vi "ma_Process RMS for 1 Block.vi"(6 "reset":bool, 7 "window for RMS":T2(ring)=enum."Hanning", 8 "time signal data (samples)":dbl[](array[numeric]) format="%0.2p", 10 "averaging type":enum16{"Linear", "Exponential"}(ring), 11 "state info":T1 {"buffer" format="%0.2f"; "timestamp" format="%<%.4X>T"; "dt history" format="%0.2f"; "t0 history" format="%<%I:%M:%S%4u %p>T"; "exp TC (samples)" format="%0.2f"; "RMS history" format="%0.2f"; "DC history" format="%0.2f"}) -> (2 "RMS value data":dbl format="%0.2f", 3 "state info":T1 {"buffer" format="%0.2f"; "timestamp" format="%<%.4X>T"; "dt history" format="%0.2f"; "t0 history" format="%<%I:%M:%S%4u %p>T"; "exp TC (samples)" format="%0.2f"; "RMS history" format="%0.2f"; "DC history" format="%0.2f"})   [LabVIEW 2022 SP3, in "NI_MAPro.lvlib"]
uses:
  NI_MAPro.lvlib
  RMS (DBL).vi
  NI_AALPro.lvlib
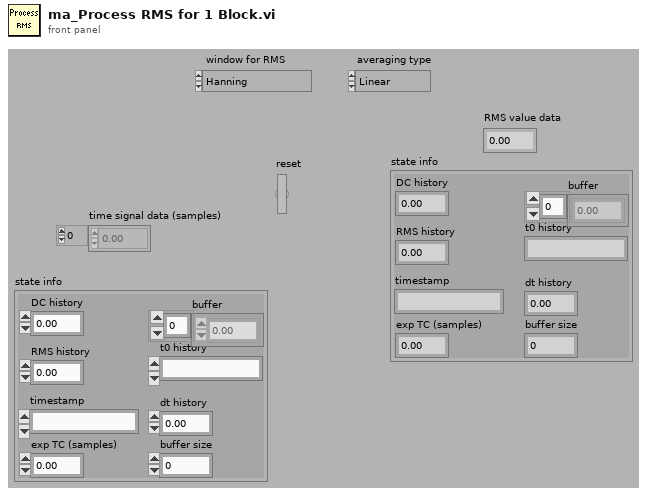
[diagram p1: front panel]
types:
  T1 = cluster{"DC history":dbl, "RMS history":dbl, "exp TC (samples)":dbl, "buffer size":i32, "t0 history":timestamp, "dt history":dbl, "timestamp":timestamp, "buffer":dbl[]}
  T2 = enum16{"Rectangular (none)", "Hanning", "Low side lobe"}
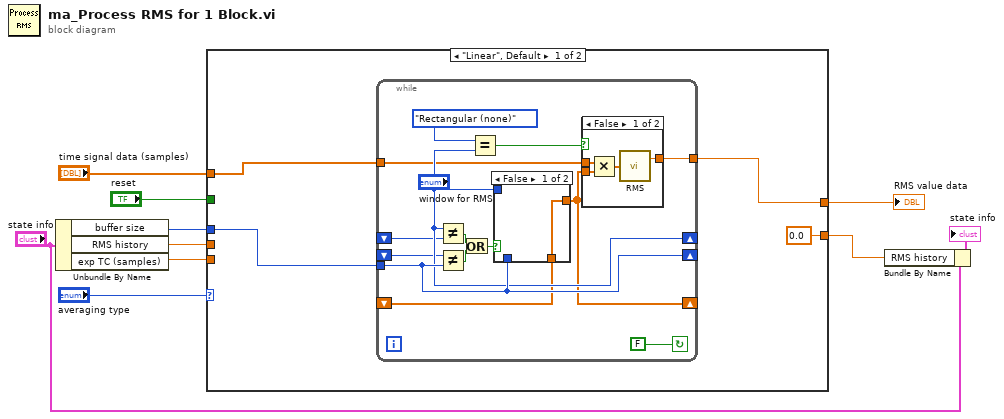
[diagram p0: block diagram]
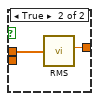
[diagram p2: hidden frame]
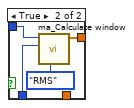
[diagram p3: hidden frame]
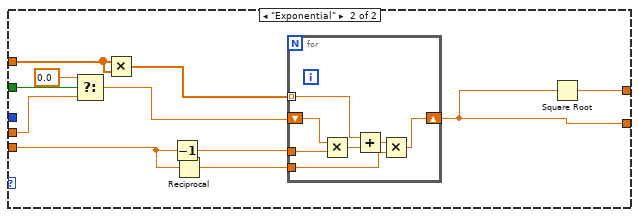
[diagram p4: hidden frame]
diagram:
  n1 = Unbundle By Name("state info") -> ("buffer size"=w6:i32, "RMS history"=w4:dbl, "exp TC (samples)"=w5:dbl)
  n2 = case shown="\"Linear\", Default" "averaging type" {
    tunnel: w6 -> [w14 _]
    tunnel: [w11 w40] -> w8
    tunnel: w5 -> [_ w48]
    tunnel: "time signal data (samples)" -> [w12 w42]
    tunnel: [0.0 w45] -> w2
    tunnel: "reset" -> [_ w44]
    tunnel: w4 -> [_ w41]
    frame "Linear", Default {
      n3 = while {
        shift-left: _ -> [w16]
        shift-right: [w19] -> _
        shift-left: _ -> [w18]
        shift-right: [w28] -> _
        shift-left: _ -> [w17]
        shift-right: ["window for RMS"] -> _
        tunnel: w12 -> [w25]
        tunnel: w14 -> [w28]
        tunnel: [w26] -> w11
        stop <- FALSE continue-if-true
        n4 = Not Equal?(x="window for RMS", y=w17) -> (x != y?=w24:bool)
        n5 = Not Equal?(x=w18, y=w28) -> (x != y?=w23:bool)
        n6 = Or(x=w24, y=w23) -> (x .or. y?=w22:bool)
        n7 = Equal?(x=T2."Rectangular (none)", y="window for RMS") -> (x = y?=w20:bool)
        n8 = case shown="False" w22 {
          tunnel: "window for RMS" -> [_ w39]
          tunnel: w28 -> [_ w38]
          tunnel: [w35 w36] -> w19
          tunnel: w16 -> [w35 _]
          frame False {
          }
          frame True {
            n9 = call "ma_Calculate window.vi"("scaled for"=enum16{"DC", "RMS"}."RMS", "array size"=w38, "window"=w39) -> ("Window data"=w36:dbl[])  [unwired: 8 in]
          }
        }
        n10 = case shown="False" w20 {
          tunnel: w25 -> [w32 w34]
          tunnel: [w31 w33] -> w26
          tunnel: w19 -> [w30 _]
          frame False {
            n11 = Multiply(x=w32, y=w30) -> (x*y=w29:dbl[])
            n12 = call-poly "RMS.vi"("X"=w29) -> ("rms value"=w31:dbl)  [unwired: 1 out]
          }
          frame True {
            n13 = call-poly "RMS.vi"("X"=w34) -> ("rms value"=w33:dbl)  [unwired: 1 out]
          }
        }
      }
    }
    frame "Exponential" {
      n14 = Select(t=0.0, s=w44, f=w41) -> (s? t:f=w49:dbl)
      n15 = Multiply(x=w42, y=w42) -> (x*y=w43:dbl[])
      n16 = Decrement(x=w48) -> (x-1=w47:dbl)
      n17 = Reciprocal(x=w48) -> (1/x=w46:dbl)
      n18 = for {
        tunnel: w43 -> [w52] mode=indexing
        shift-right: [w51] -> w45
        shift-left: w49 -> [w56]
        tunnel: w47 -> [w57]
        tunnel: w46 -> [w53]
        n19 = Multiply(x=w56, y=w57) -> (x*y=w55:dbl)
        n20 = Add(x=w52, y=w55) -> (x+y=w54:dbl)
        n21 = Multiply(x=w54, y=w53) -> (x*y=w51:dbl)
      }
      n22 = Square Root(x=w45) -> (sqrt(x)=w40:dbl)
    }
  }
  "RMS value data" <- w8
  n23 = Bundle By Name(cluster="state info", "RMS history"=w2) -> (→"state info":T1)
